vi "Recover Original Waveform from Acquired Waveform.vi"(1 "Duty Cyle Factor":dbl=2.0, 2 "A-Scan Size":i32=2000, 7 "Input Waveform":dbl[](array[numeric])) -> (8 "Recovered Waveform":dbl[](array[numeric]), 10 "Updated A-Scan Size":dbl format="%.2f", 15 "Number of A-Scans":i32)   [LabVIEW 2012]
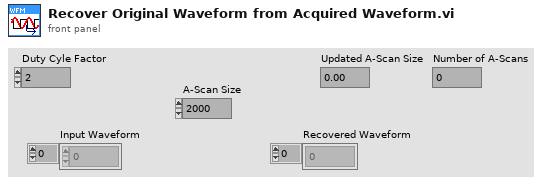
[diagram p1: front panel]
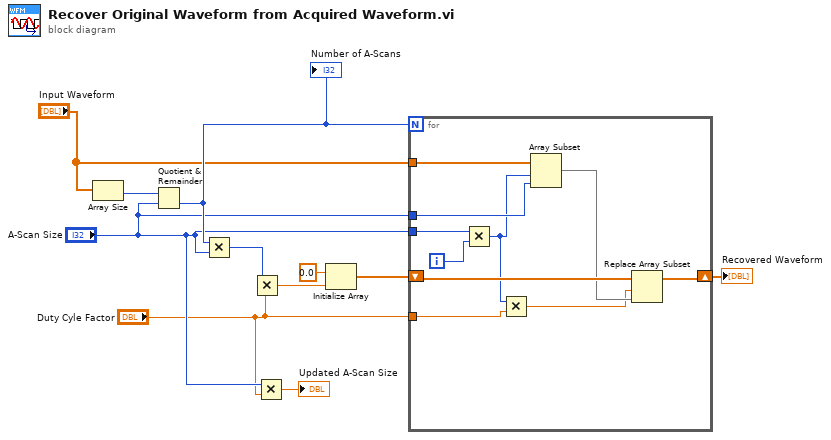
[diagram p0: block diagram]
diagram:
  n1 = Array Size(array="Input Waveform") -> (size(s)=w11:i32)
  n2 = Quotient & Remainder(x=w11, y="A-Scan Size") -> (floor(x/y)=w10:i32)  [unwired: 1 out]
  "Number of A-Scans" <- w10
  n3 = Multiply(x=w10, y="A-Scan Size") -> (x*y=w9:i32)
  n4 = Multiply(x=w9, y="Duty Cyle Factor") -> (x*y=w8:dbl)
  n5 = Multiply(x="A-Scan Size", y="Duty Cyle Factor") -> (x*y=→"Updated A-Scan Size":dbl)
  n6 = Initialize Array(0.0 ("element"), w8) -> (w6:dbl[])
  n7 = for {
    N: w10 -> [_]
    shift-right: [w12] -> w4
    shift-left: w6 -> [w21]
    tunnel: "Input Waveform" -> [w20]
    tunnel: "A-Scan Size" -> [w18]
    tunnel: "A-Scan Size" -> [w17]
    tunnel: "Duty Cyle Factor" -> [w14]
    i -> [w19]
    n8 = Multiply(x=w18, y=w19) -> (x*y=w15:i32)
    n9 = Multiply(x=w15, y=w14) -> (x*y=w13:dbl)
    n10 = Array Subset(array=w20, index=w15, length=w17) -> (w16:dbl[])
    n11 = Replace Array Subset(array=w21, new element=w16, index=w13) -> (w12:dbl[])
  }
  "Recovered Waveform" <- w4
